vi "Thermal Camera 1.vi"() -> ()   [LabVIEW 2024]
uses:
  libirimager-8.9.0-windows/irDirectSDK/examples/labview/libirimager_direct_binding.lvlib
panel:
  out "new picture":picture
  in  "stop":bool
  out "thermal_data out":u16[](array[numeric])
  out "function return thm":i32
  out "w out":i32
  out "h out":i32
  out "function return save png":i32
  in  "xml_config":string
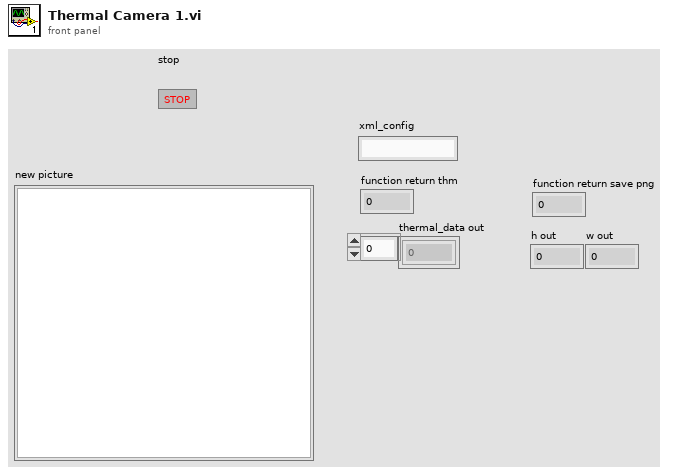
[diagram p1: front panel]
types:
  T1 = typedef "imagedata.ctl" = cluster{"image type":i32, "image depth":i32, "image":u8[], "mask":u8[], "colors":u32[], "Rectangle":cluster{"left":i16, "top":i16, "right":i16, "bottom":i16}}
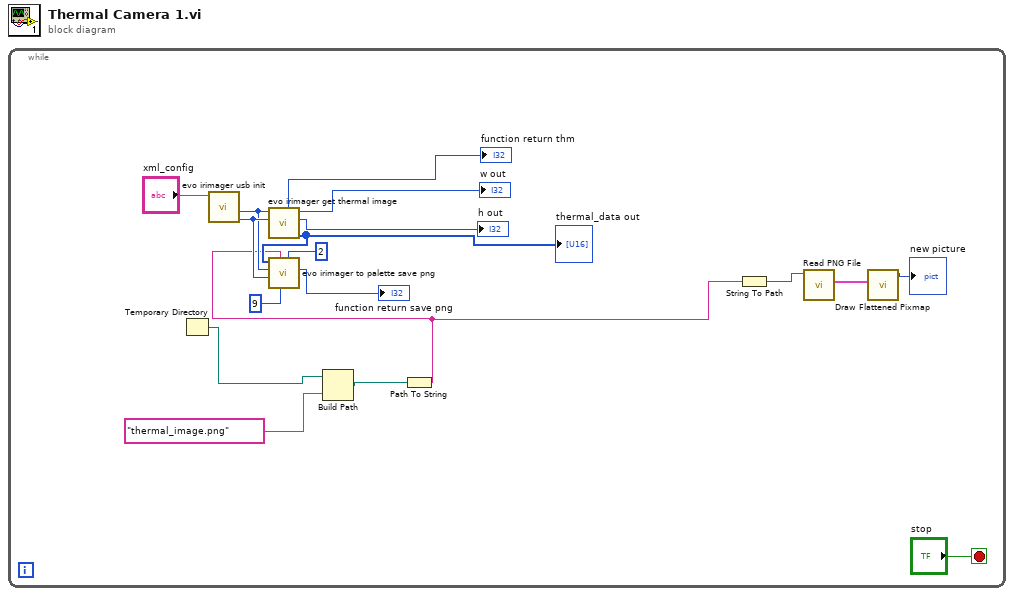
[diagram p0: block diagram]
diagram:
  n1 = while {
    stop <- "stop" stop-if-true
    n2 = Temporary Directory() -> (w7:path)
    n3 = call "evo irimager usb init.vi"("xml_config"="xml_config") -> ("h out"=w17:i32, "w out"=w16:i32)  [unwired: 7 in, 2 out]
    n4 = call "evo irimager get thermal image.vi"("h"=w17, "w"=w16) -> ("data out"=w9:u16[], "h out"=→"h out":i32, "w out"=→"w out":i32, "function return"=→"function return thm":i32)  [unwired: 6 in]
    "thermal_data out" <- w9
    n5 = Build Path(base path=w7, name or relative path="thermal_image.png" ("String")) -> (appended path=w6:path)
    n6 = Path To String(path=w6) -> (string=w4:string)
    n7 = call "evo irimager to palette save png.vi"("palette_scale"=2, "palette"=9, "path"=w4, "h"=w17, "w"=w16, "thermal_data"=w9) -> ("function return"=→"function return save png":i32)  [unwired: 4 in, 1 out]
    n8 = String To Path(string=w4) -> (path=w3:path)
    n9 = call <vilib>:"Read PNG File.vi"("path to PNG file"=w3) -> ("image data"=w2:T1)  [unwired: 8 in, 2 out]
    n10 = call <vilib>:"Draw Flattened Pixmap.vi"("image data"=w2) -> ("new picture"=→"new picture":picture)  [unwired: 8 in]
  }
